vi "update_counts.vi"(2 "Image Data In":T2, 7 "Count Display Data In":T1) -> (8 "Count Display Data Out":T1)   [LabVIEW 2023]
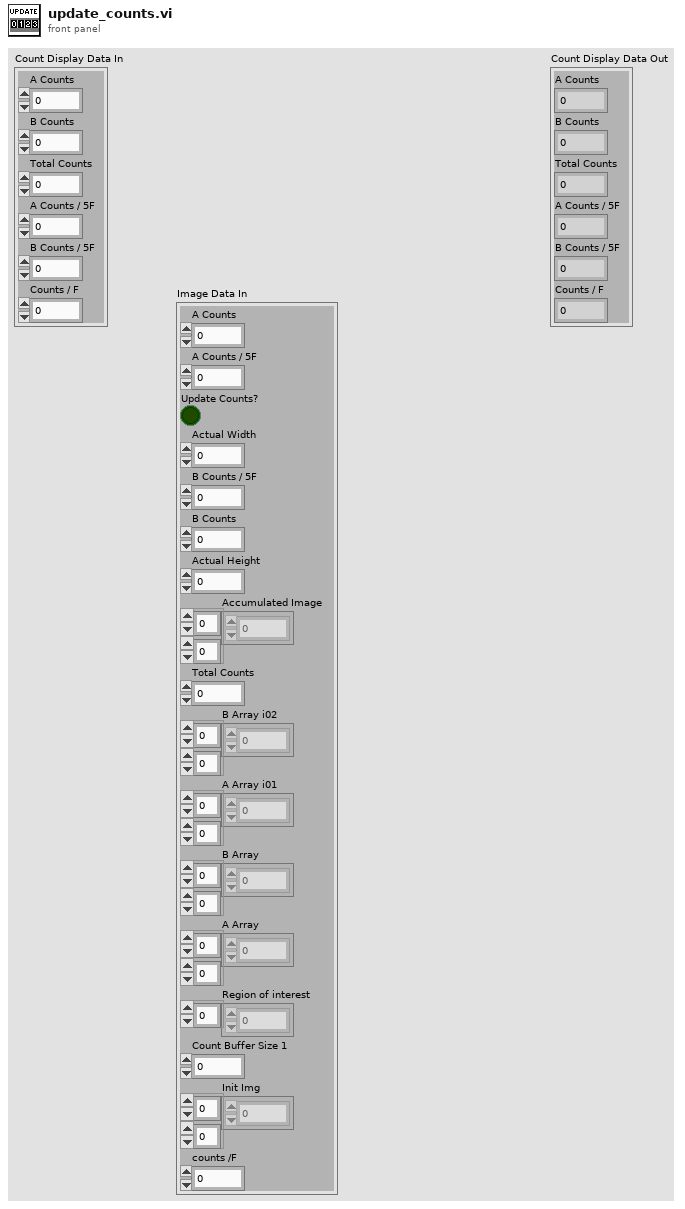
[diagram p1: front panel]
types:
  T1 = cluster{"A Counts":i32, "B Counts":i32, "Total Counts":i32, "A Counts / 5F":dbl, "B Counts / 5F":dbl, "Counts / F":dbl}
  T2 = cluster{"A Counts":i32, "A Counts / 5F":dbl, "Update Counts?":bool, "Actual Width":u32, "B Counts / 5F ":dbl, "B Counts":i32, "Actual Height":u32, "Accumulated Image ":i16[][], "Total Counts":i32, "B Array i02":sgl[][], "A Array i01":sgl[][], "B Array":i16[][], "A Array":i16[][], "Region of interest":i32[], "Count Buffer Size 1":i32, "Init Img":i16[][], "counts /F":i16}
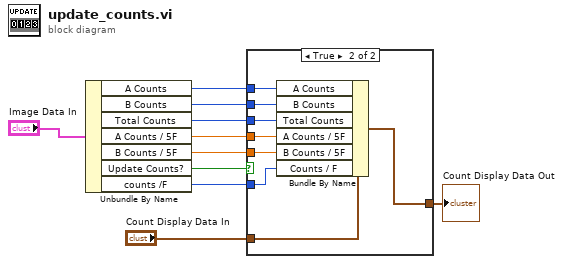
[diagram p0: block diagram]
diagram:
  n1 = Unbundle By Name("Image Data In") -> ("A Counts"=w9:i32, "B Counts"=w8:i32, "Total Counts"=w7:i32, "A Counts / 5F"=w6:dbl, "B Counts / 5F"=w5:dbl, "Update Counts?"=w10:bool, "counts /F"=w1:i16)
  n2 = case shown="True" w10 {
    tunnel: w9 -> [_ w18]
    tunnel: w8 -> [_ w17]
    tunnel: w7 -> [_ w16]
    tunnel: w6 -> [_ w15]
    tunnel: w5 -> [_ w14]
    tunnel: "Count Display Data In" -> [w11 w19]
    tunnel: [w11 w13] -> w2
    tunnel: w1 -> [_ w12]
    frame False {
    }
    frame True {
      n3 = Bundle By Name(cluster=w19, "A Counts"=w18, "B Counts"=w17, "Total Counts"=w16, "A Counts / 5F"=w15, "B Counts / 5F"=w14, "Counts / F"=w12) -> (w13:T1)
    }
  }
  "Count Display Data Out" <- w2
